vi "411x_Config.vi"(8 "error in (no error)":errorcluster, 10 "Specified Channel Ref List":T2[](array[typedef]) format="%.0x", 11 "Device Ref out":T2 format="%.0x") -> (0 "error out":errorcluster, 2 "Channel Info":T1(array[cluster]), 3 "Channel Ref List (out)":T2[](array[typedef]) format="%.0x")   [LabVIEW 2023, in "NI PXIe-411x PS Custom Device.lvlib"]
uses:
  NI PXIe-411x PS Custom Device.lvlib
  <vilib>/NI VeriStand/Custom Device API/Custom Device Item Ref.ctl
  <instrlib>/niDCPower/nidcpower.llb/niDCPower Source Mode.ctl
  <instrlib>/niDCPower/nidcpower.llb/niDCPower Output Function.ctl
  411x_Global.vi
  <vilib>/NI VeriStand/Custom Device API/Get Item Property (String).vi
  <vilib>/NI VeriStand/Custom Device API/Get Item Property (U16).vi
  <vilib>/NI VeriStand/Custom Device API/Get Item Property (I32).vi
  <vilib>/NI VeriStand/Custom Device API/Get Item Property (Double).vi
  <vilib>/NI VeriStand/Custom Device API/Get Item Property (Boolean).vi
  <vilib>/NI VeriStand/Custom Device API/Custom Device API.lvlib
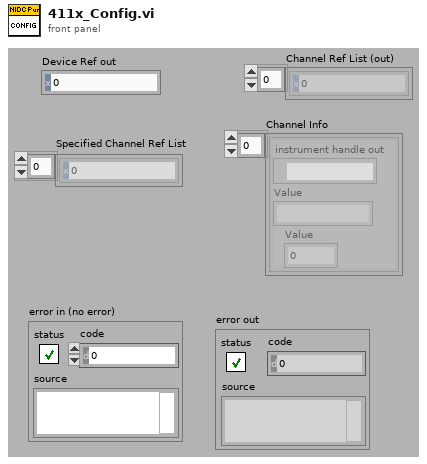
[diagram p1: front panel]
types:
  T1 = cluster{"instrument handle out":refnum<k15>, "Value":string, "Value":u16}[]
  T2 = typedef "Custom Device API.lvlib/Custom Device Item Ref.ctl" = u64
  T3 = typedef "niDCPower Source Mode.ctl" = i32
  T4 = typedef "niDCPower Output Function.ctl" = i32
  T5 = cluster{"instrument handle out":refnum<k15>, string, "Value":u16}
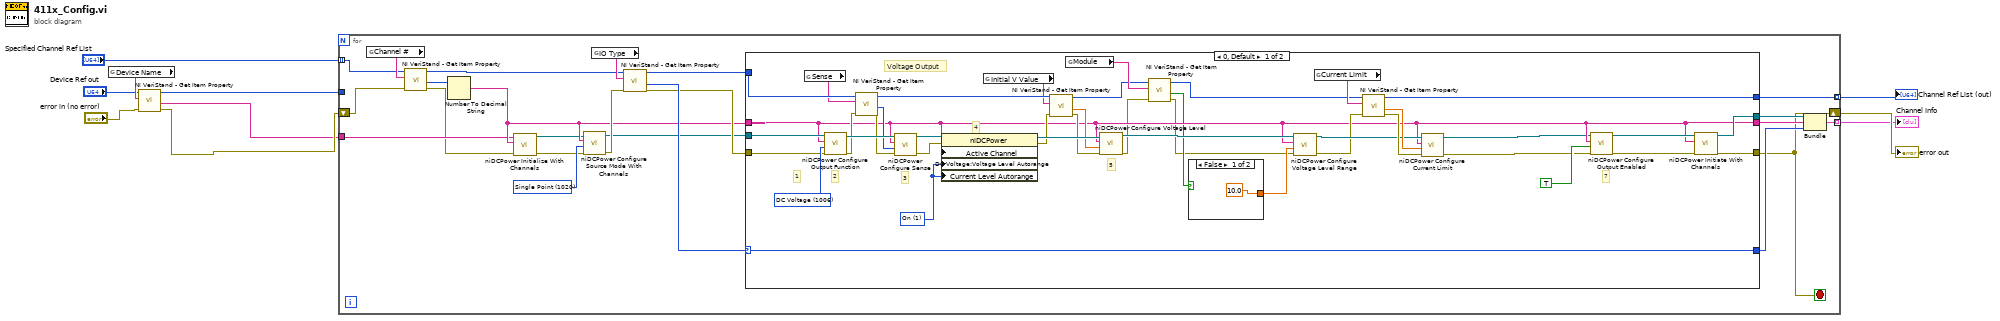
[diagram p0: block diagram]
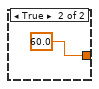
[diagram p2: hidden frame]
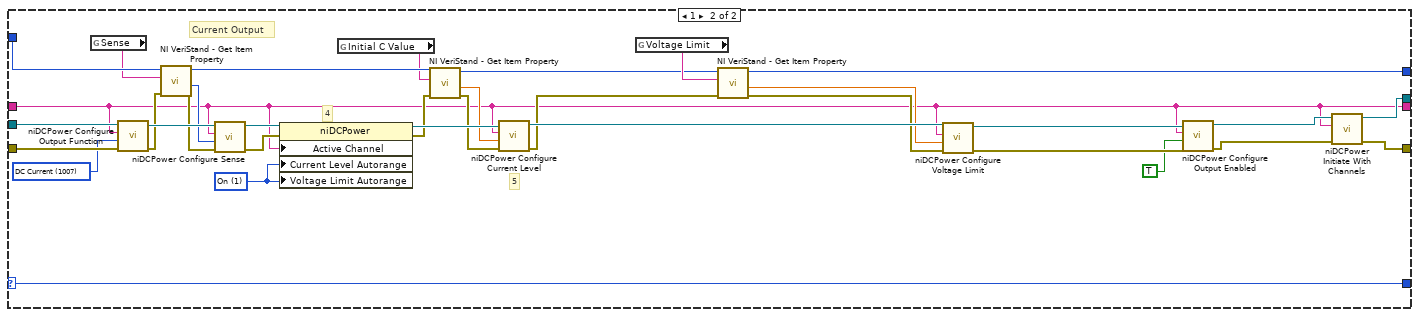
[diagram p3: hidden frame]
diagram:
  n1 = global read "411x_Global.vi" "Device Name"() -> (w8:string)
  n2 = call-poly <vilib>:"NI VeriStand - Get Item Property.vi"("error in (no error)"="error in (no error)", "Property Name"=w8, "Item Ref in"="Device Ref out") -> ("error out"=w2:errorcluster, "Value"=w1:string, "Item Ref out"=w5:T2)  [unwired: 5 in, 1 out]
  n3 = for {
    tunnel: "Specified Channel Ref List" -> [w21] mode=indexing
    tunnel: [w33] -> w3 mode=indexing
    tunnel: w5 -> [_]
    tunnel: [w28] -> w4 mode=indexing
    shift-right: [w26] -> w9
    shift-left: w2 -> [w18]
    tunnel: w1 -> [w14]
    stop <- w26 stop-if-true
    w19 = T3 1020 items=["Single Point"=1020, "Sequence"=1021] ("source mode")
    n4 = global read "411x_Global.vi" "Channel #"() -> (w23:string)
    n5 = call-poly <vilib>:"NI VeriStand - Get Item Property.vi"("error in (no error)"=w18, "Property Name"=w23, "Item Ref in"=w21) -> ("error out"=w13:errorcluster, "Value"=w22:u16, "Item Ref out"=w20:T2)  [unwired: 5 in, 1 out]
    n6 = Number To Decimal String(number=w22) -> (decimal integer string=w15:string)  [unwired: 1 in]
    n7 = call <instrlib>:"niDCPower Initialize With Channels.vi"("error in (no error)"=w13, "channels"=w15, "resource name"=w14) -> ("error out"=w12:errorcluster, "instrument handle out"=w11:refnum<k15>)  [unwired: 7 in]
    n8 = call <instrlib>:"niDCPower Configure Source Mode With Channels.vi"("error in (no error)"=w12, "source mode"=w19, "channel name"=w15, "instrument handle"=w11) -> ("error out"=w17:errorcluster, "instrument handle out"=w16:refnum<k15>)  [unwired: 6 in]
    n9 = global read "411x_Global.vi" "IO Type"() -> (w30:string)
    n10 = call-poly <vilib>:"NI VeriStand - Get Item Property.vi"("error in (no error)"=w17, "Property Name"=w30, "Item Ref in"=w20) -> ("error out"=w24:errorcluster, "Value"=w29:u16, "Item Ref out"=w25:T2)  [unwired: 5 in, 1 out]
    n11 = case shown="0, Default" w29 {
      selector: w29 -> [w53 w87]
      tunnel: [w46 w77] -> w26
      tunnel: [w45 w80] -> w32
      tunnel: [w44 w79] -> w31
      tunnel: w16 -> [w69 w103]
      tunnel: w25 -> [w68 w102]
      tunnel: w15 -> [w44 w79]
      tunnel: w24 -> [w65 w99]
      tunnel: [w54 w88] -> w28
      tunnel: [w53 w87] -> w27
      frame 0, Default {
        w74 = T4 1006 items=["DC Voltage"=1006, "DC Current"=1007] ("output function")
        w36 = 1 items=["Off", "On"] ("DC Voltage:Voltage Level Autorange")
        # "Voltage Output"
        # "7"
        # "5"
        # "2"
        # "4"
        # "3"
        # "1"
        n12 = global read "411x_Global.vi" "Sense"() -> (w67:string)
        n13 = call <instrlib>:"niDCPower Configure Output Function.vi"("error in (no error)"=w65, "output function"=w74, "channel name"=w44, "instrument handle"=w69) -> ("error out"=w64:errorcluster, "instrument handle out"=w73:refnum<k15>)  [unwired: 6 out]
        n14 = call-poly <vilib>:"NI VeriStand - Get Item Property.vi"("error in (no error)"=w64, "Property Name"=w67, "Item Ref in"=w68) -> ("error out"=w63:errorcluster, "Value"=w66:i32, "Item Ref out"=w62:T2)  [unwired: 5 in, 1 out]
        n15 = call <instrlib>:"niDCPower Configure Sense.vi"("error in (no error)"=w63, "sense"=w66, "channel name"=w44, "instrument handle"=w73) -> ("error out"=w72:errorcluster, "instrument handle out"=w70:refnum<k15>)  [unwired: 6 out]
        n16 = property class="niDCPower"(reference=w70, error in=w72, "Active Channel"=w44, "DC Voltage:Voltage Level Autorange"=w36, "Current Level Autorange"=w36) -> (reference out=w71:refnum<k15>, error out=w60:errorcluster)
        n17 = global read "411x_Global.vi" "Initial V Value"() -> (w61:string)
        n18 = call-poly <vilib>:"NI VeriStand - Get Item Property.vi"("error in (no error)"=w60, "Property Name"=w61, "Item Ref in"=w62) -> ("error out"=w59:errorcluster, "Value"=w58:dbl, "Item Ref out"=w42:T2)  [unwired: 5 in, 1 out]
        n19 = global read "411x_Global.vi" "Module"() -> (w43:string)
        n20 = call <instrlib>:"niDCPower Configure Voltage Level.vi"("error in (no error)"=w59, "voltage level"=w58, "channel name"=w44, "instrument handle"=w71) -> ("error out"=w38:errorcluster, "instrument handle out"=w52:refnum<k15>)  [unwired: 6 out]
        n21 = call-poly <vilib>:"NI VeriStand - Get Item Property.vi"("error in (no error)"=w38, "Property Name"=w43, "Item Ref in"=w42) -> ("error out"=w37:errorcluster, "Value"=w39:bool, "Item Ref out"=w41:T2)  [unwired: 5 in, 1 out]
        n22 = case shown="False" w39 {
          tunnel: [10.0 ("voltage level range") 60.0 ("voltage level range")] -> w40
          frame False {
          }
          frame True {
          }
        }
        n23 = call <instrlib>:"niDCPower Configure Voltage Level Range.vi"("error in (no error)"=w37, "voltage level range"=w40, "channel name"=w44, "instrument handle"=w52) -> ("error out"=w50:errorcluster, "instrument handle out"=w51:refnum<k15>)  [unwired: 6 in]
        n24 = global read "411x_Global.vi" "Current Limit"() -> (w57:string)
        n25 = call-poly <vilib>:"NI VeriStand - Get Item Property.vi"("error in (no error)"=w50, "Property Name"=w57, "Item Ref in"=w41) -> ("error out"=w56:errorcluster, "Value"=w55:dbl, "Item Ref out"=w54:T2)  [unwired: 5 in, 1 out]
        n26 = call <instrlib>:"niDCPower Configure Current Limit.vi"("error in (no error)"=w56, "current limit"=w55, "channel name"=w44, "instrument handle"=w51) -> ("error out"=w34:errorcluster, "instrument handle out"=w35:refnum<k15>)  [unwired: 1 in, 5 out]
        n27 = call <instrlib>:"niDCPower Configure Output Enabled.vi"("error in (no error)"=w34, "output enabled"=TRUE, "channel name"=w44, "instrument handle"=w35) -> ("error out"=w47:errorcluster, "instrument handle out"=w48:refnum<k15>)  [unwired: 6 out]
        n28 = call <instrlib>:"niDCPower Initiate With Channels.vi"("error in (no error)"=w47, "channel name"=w44, "instrument handle"=w48) -> ("error out"=w46:errorcluster, "instrument handle out"=w45:refnum<k15>)  [unwired: 7 in]
      }
      frame 1 {
        w83 = T4 1007 items=["DC Voltage"=1006, "DC Current"=1007] ("output function")
        w84 = 1 items=["Off", "On"] ("DC Voltage:Voltage Level Autorange")
        # "Current Output"
        # "5"
        # "4"
        n29 = global read "411x_Global.vi" "Sense"() -> (w101:string)
        n30 = call <instrlib>:"niDCPower Configure Output Function.vi"("error in (no error)"=w99, "output function"=w83, "channel name"=w79, "instrument handle"=w103) -> ("error out"=w98:errorcluster, "instrument handle out"=w110:refnum<k15>)  [unwired: 6 out]
        n31 = call-poly <vilib>:"NI VeriStand - Get Item Property.vi"("error in (no error)"=w98, "Property Name"=w101, "Item Ref in"=w102) -> ("error out"=w97:errorcluster, "Value"=w100:i32, "Item Ref out"=w96:T2)  [unwired: 5 in, 1 out]
        n32 = call <instrlib>:"niDCPower Configure Sense.vi"("error in (no error)"=w97, "sense"=w100, "channel name"=w79, "instrument handle"=w110) -> ("error out"=w109:errorcluster, "instrument handle out"=w104:refnum<k15>)  [unwired: 6 out]
        n33 = property class="niDCPower"(reference=w104, error in=w109, "Active Channel"=w79, "Current Level Autorange"=w84, "Voltage Limit Autorange"=w84) -> (reference out=w108:refnum<k15>, error out=w94:errorcluster)
        n34 = global read "411x_Global.vi" "Initial C Value"() -> (w95:string)
        n35 = call-poly <vilib>:"NI VeriStand - Get Item Property.vi"("error in (no error)"=w94, "Property Name"=w95, "Item Ref in"=w96) -> ("error out"=w93:errorcluster, "Value"=w85:dbl, "Item Ref out"=w86:T2)  [unwired: 5 in, 1 out]
        n36 = call <instrlib>:"niDCPower Configure Current Level.vi"("error in (no error)"=w93, "current level"=w85, "channel name"=w79, "instrument handle"=w108) -> ("error out"=w91:errorcluster, "instrument handle out"=w107:refnum<k15>)  [unwired: 6 in]
        n37 = global read "411x_Global.vi" "Voltage Limit"() -> (w92:string)
        n38 = call-poly <vilib>:"NI VeriStand - Get Item Property.vi"("error in (no error)"=w91, "Property Name"=w92, "Item Ref in"=w86) -> ("error out"=w90:errorcluster, "Value"=w89:dbl, "Item Ref out"=w88:T2)  [unwired: 5 in, 1 out]
        n39 = call <instrlib>:"niDCPower Configure Voltage Limit.vi"("error in (no error)"=w90, "voltage limit"=w89, "channel name"=w79, "instrument handle"=w107) -> ("error out"=w105:errorcluster, "instrument handle out"=w106:refnum<k15>)  [unwired: 6 in]
        n40 = call <instrlib>:"niDCPower Configure Output Enabled.vi"("error in (no error)"=w105, "output enabled"=TRUE ("Output Enabled"), "channel name"=w79, "instrument handle"=w106) -> ("error out"=w78:errorcluster, "instrument handle out"=w81:refnum<k15>)  [unwired: 6 out]
        n41 = call <instrlib>:"niDCPower Initiate With Channels.vi"("error in (no error)"=w78, "channel name"=w79, "instrument handle"=w81) -> ("error out"=w77:errorcluster, "instrument handle out"=w80:refnum<k15>)  [unwired: 7 in]
      }
    }
    n42 = Bundle("instrument handle out"=w32, w31, "Value"=w27) -> (w33:T5)  [unwired: 1 in]
  }
  "error out" <- w9
  "Channel Ref List (out)" <- w4
  "Channel Info" <- w3
